vi "JSON to CSV.vi"(9 "Zones":T1[](array[typedef]), 10 "CSV File":path, 11 "JSON Path":path) -> ()   [LabVIEW 2015]
uses:
  Typedef/Zone Data.ctl
  <vilib>/Utility/file.llb/Write Delimited Spreadsheet (string).vi
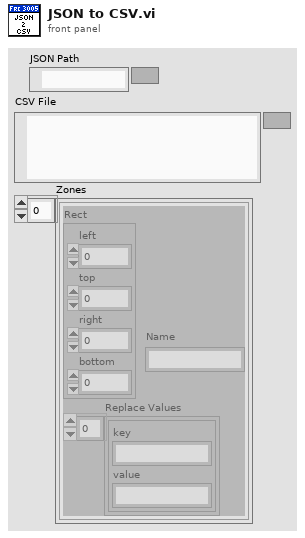
[diagram p1: front panel]
types:
  T1 = typedef "Zone Data.ctl" = cluster{"Rect":cluster{"left":i16, "top":i16, "right":i16, "bottom":i16}, "Replace Values":cluster{"key":string, "value":string}[], "Name":string}
  T2 = typedef "JSONCluster.ctl" = cluster{"preMatchData":cluster{"teamNumber":i32, "matchNumber":i32, "defenses":cluster{"blue1":string, "blue2":string, "blue3":string, "blue4":string, "blue5":string, "red1":string, "red2":string, "red3":string, "red4":string, "red5":string}}, "matchData":cluster{"name":string, "items":cluster{"x":i32, "y":i32, "value":string}[]}[], "matchComments":cluster{"matchComments":string, "lastComments":string}}
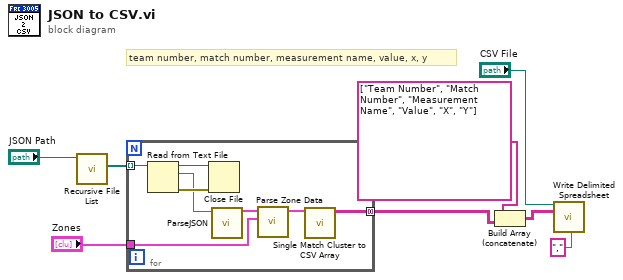
[diagram p0: block diagram]
diagram:
  # "team number, match number, measurement name, value, x, y"
  n1 = call <vilib>:"Recursive File List.vi"("Folder Path"="JSON Path") -> ("All Files in Dir"=w8:path[])  [unwired: 6 in, 4 out]
  n2 = for {
    tunnel: w8 -> [w16] mode=indexing
    tunnel: [w12] -> w4 mode=concatenating
    tunnel: "Zones" -> [w9]
    n3 = Read from Text File(file (use dialog)=w16) -> (refnum out=w14:refnum<file>, text=w13:string, error out=w15:errorcluster)  [unwired: 3 in, 1 out]
    n4 = Close File(refnum=w14, error in=w15) -> ()  [unwired: 2 out]
    n5 = call "ParseJSON.vi"("JSON String"=w13) -> ("JSONCluster"=w11:T2)  [unwired: 9 in, 1 out]
    n6 = call "Parse Zone Data.vi"("Zones"=w9, "JSONCluster in"=w11) -> ("JSONCluster out"=w10:T2)  [unwired: 9 in]
    n7 = call "Single Match Cluster to CSV Array.vi"("Match Cluster"=w10) -> ("csv array"=w12:string[][])  [unwired: 10 in]
  }
  n8 = Build Array (concatenate)(string[] ["Team Number", "Match Number", "Measurement Name", "Value", "X", "Y"], w4) -> (w2:string[][])
  n9 = call-poly <vilib>:"Write Delimited Spreadsheet.vi"("file path (dialog if empty)"="CSV File", "2D data"=w2, "delimiter (\\t)"="," ("delimiter (\\t)")) -> ()  [unwired: 11 in, 2 out]
